vi "Calculate Angle.vi"(10 "Current Angle":dbl, 11 "Target Angle":dbl) -> (2 "Clockwise":bool, 3 "Delta Angle":dbl)   [LabVIEW 2015]
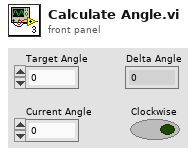
[diagram p1: front panel]
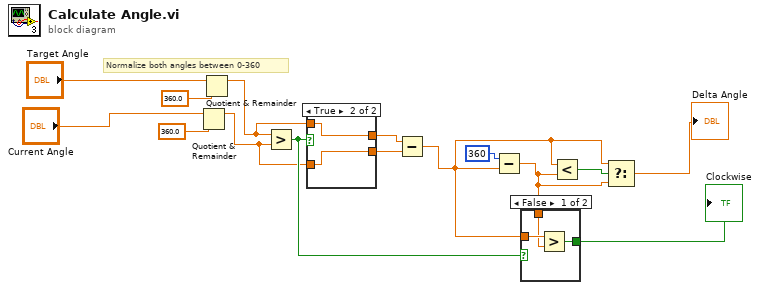
[diagram p0: block diagram]
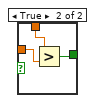
[diagram p2: hidden frame]
diagram:
  # "Normalize both angles between 0-360"
  n1 = Quotient & Remainder(x="Current Angle", y=360.0) -> (x-y*floor(x/y)=w8:dbl)  [unwired: 1 out]
  n2 = Quotient & Remainder(x="Target Angle", y=360.0) -> (x-y*floor(x/y)=w7:dbl)  [unwired: 1 out]
  n3 = Greater?(x=w7, y=w8) -> (0:w12:bool)
  n4 = case shown="True" w12 {
    tunnel: [w17 w19] -> w5
    tunnel: [w16 w18] -> w6
    tunnel: w7 -> [w16 w19]
    tunnel: w8 -> [w17 w18]
    frame False {
    }
    frame True {
    }
  }
  n5 = Subtract(x=w5, y=w6) -> (x-y=w13:dbl)
  n6 = Subtract(x=360, y=w13) -> (x-y=w14:dbl)
  n7 = case shown="False" w12 {
    tunnel: w13 -> [w22 w25]
    tunnel: w14 -> [w21 w24]
    tunnel: [w20 w23] -> w15
    frame False {
      n8 = Greater?(x=w22, y=w21) -> (0:w20:bool)
    }
    frame True {
      n9 = Greater?(x=w24, y=w25) -> (0:w23:bool)
    }
  }
  "Clockwise" <- w15
  n10 = Less?(x=w13, y=w14) -> (x < y?=w10:bool)
  n11 = Select(t=w13, s=w10, f=w14) -> (s? t:f=→"Delta Angle":dbl)
